vi "initialize debug mode.vi"(10 "User Event in":T1, 11 "editor node in":T2) -> (1 "engine":refnum<data-value>, 2 "User Event out":T1, 3 "editor node out":T2, 5 "Engine Configuration":refnum<class "engine configuration.lvclass">)   [LabVIEW 2013, in "configuration tests.lvlib" / "TEST EDITOR.lvclass"]
uses:
  TEST EDITOR.lvclass
  <vilib>/CEF_TreeControl/Node/NodeRef.ctl
  <vilib>/CEF_TreeControl/Node/NISE_CEF_Node.lvclass
  Configuration Editor/Classes/Engine Parent/Engine Parent Editor Node.lvclass
  <vilib>/CEF_TreeControl/Node/UserEventRef.ctl
  <vilib>/CEF_TreeControl/Controls/EventCluster.ctl
  <vilib>/NI/Module Execution Interface/Engine Configuration/engine configuration.lvclass
  module/configuration/TEST CONFIGURATION.lvclass
  <vilib>/NI/Tag Bus/tag/Data Type.ctl
  <vilib>/NI/Tag Bus/tag/tag descriptor.lvclass/tag descriptor.ctl
  Configuration Editor/Classes/Engine Parent/read engine configuration.vi
  Configuration Editor/Classes/Engine Parent/write engine configuration.vi
  <vilib>/NI/Tag Bus/tag/tag descriptor.lvclass
  <vilib>/CEF_TreeControl/NISE_CEF_TreeControl.lvlib
  Configuration Editor/Classes/Module editor node/module editor node.lvclass
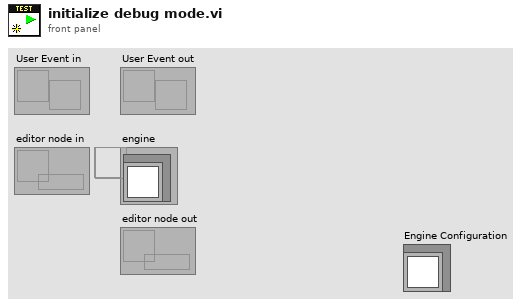
[diagram p1: front panel]
types:
  T1 = typedef "NISE_CEF_Node.lvclass/UserEventRef.ctl" = refnum<user-event>
  T2 = typedef "NISE_CEF_Node.lvclass/NodeRef.ctl" = refnum<data-value>
  T3 = typedef "NISE_CEF_TreeControl.lvlib/EventCluster.ctl" = cluster{"command":string, "data":string}
  T4 = typedef "tag bus.lvlib/tag descriptor.lvclass/Data Type.ctl" = enum16{"Double", "Single", "I64", "I32", "I16", "I8", "U64", "U32", "U16", "U8", "Boolean", "String", "Array of Double", "Array of Single", "Array of I64", "Array of I32", "Array of I16", "Array of I8", "Array of U64", "Array of U32", "Array of U16", "Array of U8", "Array of Boolean", "Array of String"}
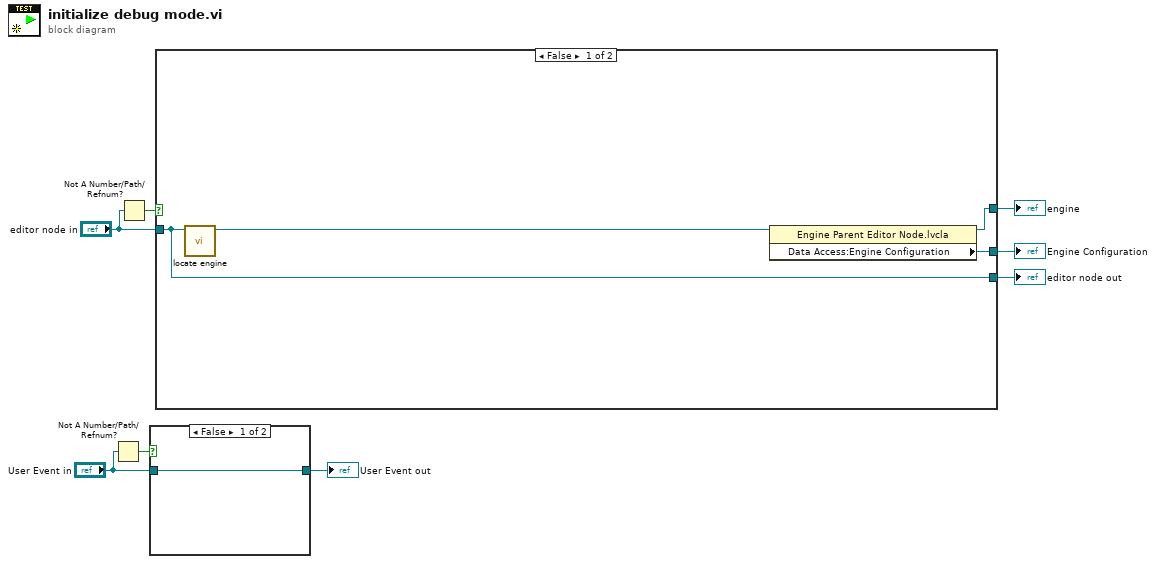
[diagram p0: block diagram]
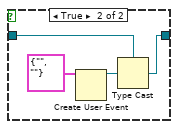
[diagram p2: hidden frame]
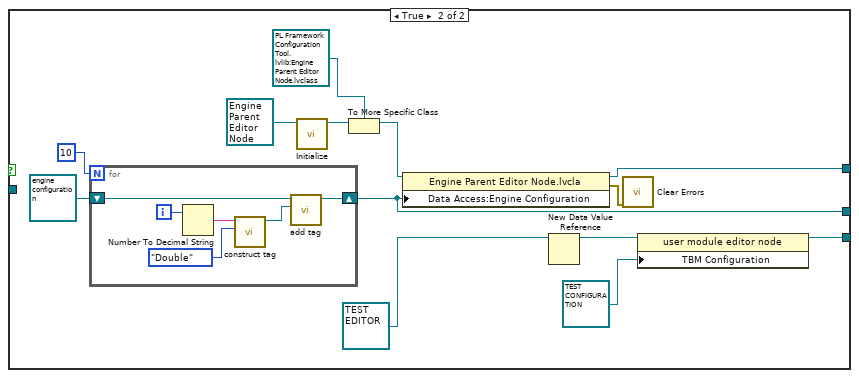
[diagram p3: hidden frame]
diagram:
  n1 = Not A Number/Path/Refnum?(number/path/refnum="User Event in") -> (NaN/Path/Refnum?=w4:bool)
  n2 = Not A Number/Path/Refnum?(number/path/refnum="editor node in") -> (NaN/Path/Refnum?=w5:bool)
  n3 = case shown="False" w4 {
    tunnel: "User Event in" -> [w9 w10]
    tunnel: [w9 w11] -> w2
    frame False {
    }
    frame True {
      n4 = Create User Event(user event datatype=T3 {"command"="", "data"=""} ("event data")) -> (user event=w12:refnum<user-event>)  [unwired: 1 in, 1 out]
      n5 = Type Cast(type=w10, x=w12) -> (*(type *) &x=w11:T1)
    }
  }
  "User Event out" <- w2
  n6 = case shown="False" w5 {
    tunnel: "editor node in" -> [w16 _]
    tunnel: [w16 w30] -> w7
    tunnel: [w15 w22] -> w6
    tunnel: [w14 w20] -> w1
    frame False {
      n7 = call "locate engine.vi"("component"=w16) -> ("engine"=w17:refnum<data-value>)  [unwired: 9 in, 1 out]
      n8 = property class="Engine Parent Editor Node.lvcla"(reference=w17) -> (reference out=w15:refnum<data-value>, "Data Access:Engine Configuration"=w14:refnum<class "engine configuration.lvclass">)  [unwired: 1 in, 1 out]
    }
    frame True {
      n9 = for {
        N: 10 -> [_]
        shift-right: [w35] -> w20
        shift-left: refnum<class "engine configuration.lvclass"> refnum ("Engine Configuration") -> [w36]
        i -> [w33]
        n10 = Number To Decimal String(number=w33) -> (decimal integer string=w32:string)  [unwired: 1 in]
        n11 = call <vilib>:"construct tag.vi"("data type"=Data_Type."Double", "name"=w32) -> ("system tag out"=w34:refnum<class "tag descriptor.lvclass">)  [unwired: 9 in]
        n12 = call <vilib>:"add tag.vi"("tag descriptor"=w34, "engine configuration in"=w36) -> ("engine configuration out"=w35:refnum<class "engine configuration.lvclass">)  [unwired: 8 in, 1 out]
      }
      n13 = call-dynamic "Initialize.vi"("Engine in"=refnum<class "Engine Parent Editor Node.lvclass"> refnum ("PL Framework Configuration Tool.lvlib:Engine Parent Editor Node.lvclass")) -> ("data value reference"=w29:T2)  [unwired: 8 in, 2 out]
      n14 = To More Specific Class(target class=refnum<data-value> refnum ("data value reference"), reference=w29) -> (specific class reference=w28:refnum<data-value>)  [unwired: 1 in, 1 out]
      n15 = property class="Engine Parent Editor Node.lvcla"(reference=w28, "Data Access:Engine Configuration"=w20) -> (reference out=w22:refnum<data-value>, error out=w18:errorcluster)  [unwired: 1 in]
      n16 = New Data Value Reference(data value=refnum<class "TEST EDITOR.lvclass"> refnum ("tag bus configurable plugin editor node")) -> (data value reference=w26:refnum<data-value>)  [unwired: 1 in, 1 out]
      n17 = call <vilib>:"Clear Errors.vi"("error in (no error)"=w18) -> ()  [unwired: 6 in, 1 out]
      n18 = property class="user module editor node"(reference=w26, "TBM Configuration"=refnum<class "TEST CONFIGURATION.lvclass"> refnum ("user module configuration")) -> (reference out=w30:refnum<data-value>)  [unwired: 1 in, 1 out]
    }
  }
  "editor node out" <- w7
  "engine" <- w6
  "Engine Configuration" <- w1
